vi "MidiSetup.vi"(8 "error in (no error)":errorcluster, 10 "CtrlC":bool, 11 "hub":string) -> (0 "error out":errorcluster, 2 "guess":string, 3 "Python":T1)   [LabVIEW 2022 SP3]
uses:
  PythonCtrl.ctl
  Processors.ctl
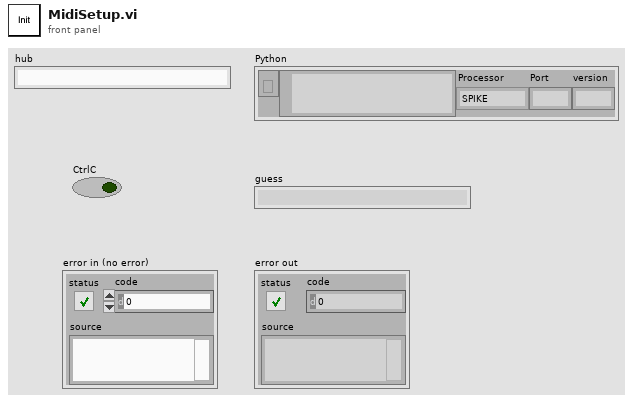
[diagram p1: front panel]
types:
  T1 = typedef "PythonCtrl.ctl" = cluster{"session":refnum<k35>, "PyPath":path, "Processor":T2, "Port":string, "version":string}
  T2 = typedef "Processors.ctl" = enum16{"SPIKE", "Pi", "Pi_ssh", "OpenMV", "Dunio"}
  T3 = typedef "Preferences.ctl" = cluster{"python":string, "arduino CLI":path, "pythonCodes":cluster{"pythonCode":path, "Color":u32}[], "FontSize":u8, "Text Colors":cluster{"Quote":u32, "function":u32, "Python":u32, "Comment":u32, "Triple Quote":u32, "Text":u32}, "SSH Logins":cluster{"IP Address":string, "Username":string, "password":string}[]}
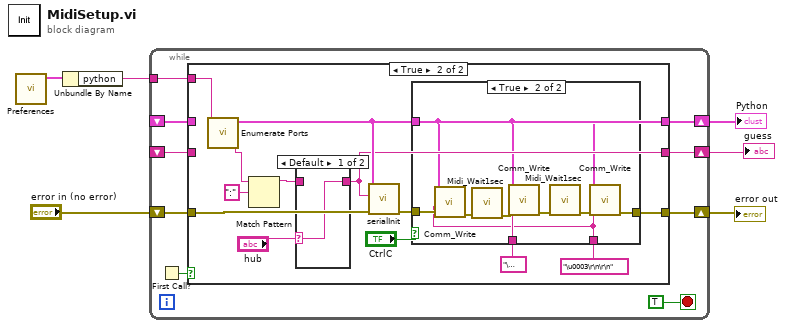
[diagram p0: block diagram]
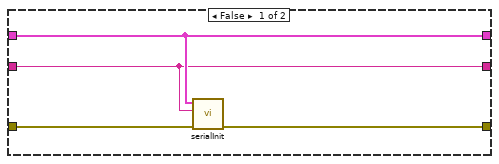
[diagram p2: hidden frame]
diagram:
  n1 = call "Preferences.vi"() -> ("Preferences out"=w2:T3)  [unwired: 10 in, 1 out]
  n2 = Unbundle By Name(w2) -> ("python"=w1:string)
  n3 = while {
    shift-right: [w14] -> w5
    shift-left: "error in (no error)" -> [w15]
    shift-right: [w12] -> w4
    shift-left: _ -> [w10]
    shift-right: [w9] -> w3
    shift-left: _ -> [w8]
    tunnel: w1 -> [w7]
    stop <- TRUE stop-if-true
    n4 = First Call?() -> (First Call?: T/F=w11:bool)
    n5 = case shown="True" w11 {
      tunnel: w15 -> [w16 w32]
      tunnel: [w17 w31] -> w14
      tunnel: [w19 w27] -> w12
      tunnel: w10 -> [w19 _]
      tunnel: [w18 w22] -> w9
      tunnel: w8 -> [w18 _]
      tunnel: w7 -> [_ w24]
      frame False {
        n6 = call "serialInit.vi"("error in (no error)"=w16, "Port"=w18, "Python"=w19) -> ("error out"=w17:errorcluster)  [unwired: 6 in, 2 out]
      }
      frame True {
        n7 = call "Enumerate Ports.vi"("Python version"=w24) -> ("guess"=w26:string, "Python"=w27:T1)  [unwired: 6 in, 3 out]
        n8 = Match Pattern(string=w26, regular expression=":") -> (before substring=w21:string)  [unwired: 1 in, 3 out]
        n9 = case shown="Default" "hub" {
          selector: "hub" -> [w33 _]
          tunnel: [w33 w34] -> w22
          tunnel: w21 -> [_ w34]
          frame Default {
          }
          frame "" {
          }
        }
        n10 = call "serialInit.vi"("error in (no error)"=w32, "Port"=w22, "Python"=w27) -> ("error out"=w29:errorcluster)  [unwired: 6 in, 2 out]
        n11 = case shown="True" "CtrlC" {
          tunnel: w29 -> [w35 w40]
          tunnel: "\u0003\r\n\r\n" ("function name") -> [_ w36]
          tunnel: w27 -> [_ w37]
          tunnel: [w35 w44] -> w31
          tunnel: "\u0004" ("function name") -> [_ w43]
          frame False {
          }
          frame True {
            n12 = call "Comm_Write.vi"("error in (no error)"=w40, "Text to write"=w36, "Python"=w37) -> ("error out"=w39:errorcluster)  [unwired: 7 in, 1 out]
            n13 = call "Midi_Wait1sec.vi"("error in (no error)"=w39) -> ("error out"=w38:errorcluster)  [unwired: 10 in]
            n14 = call "Comm_Write.vi"("error in (no error)"=w38, "Text to write"=w43, "Python"=w37) -> ("error out"=w42:errorcluster)  [unwired: 7 in, 1 out]
            n15 = call "Midi_Wait1sec.vi"("error in (no error)"=w42) -> ("error out"=w41:errorcluster)  [unwired: 10 in]
            n16 = call "Comm_Write.vi"("error in (no error)"=w41, "Text to write"=w36, "Python"=w37) -> ("error out"=w44:errorcluster)  [unwired: 7 in, 1 out]
          }
        }
      }
    }
  }
  "error out" <- w5
  "Python" <- w4
  "guess" <- w3
